vi "Host API Example.vi"() -> ()   [LabVIEW 2013]
uses:
  Shared/Types/Update Parameters Message.ctl
  Shared/Types/Get Settings Message.ctl
  Shared/Types/Gain Schedule.ctl
  Host API/PID Control Host API.lvlib
  Shared/Control Addon Shared.lvlib
panel:
  out "Timed Out?":bool
  out "Settings":T1
  in  "Parameters":T3
  in  "Apply":bool
  in  "Stop":bool
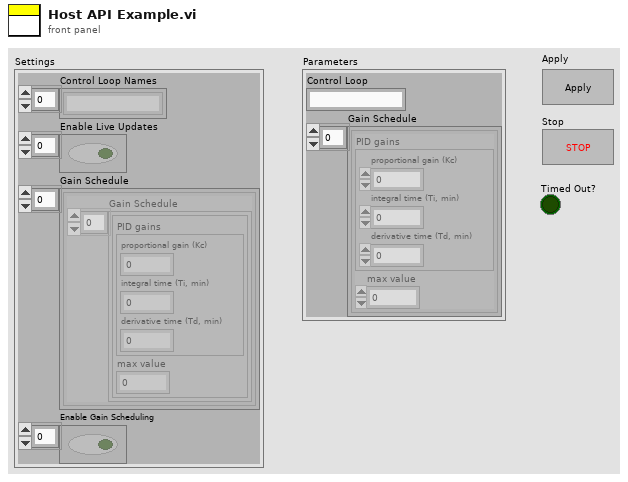
[diagram p1: front panel]
types:
  T1 = typedef "Control Addon Shared.lvlib/Get Settings Message.ctl" = cluster{"Control Loop Names":string[], "Enable Live Updates":bool[], "Gain Schedule":T2[], "Enable Gain Scheduling":bool[]}
  T2 = typedef "Control Addon Shared.lvlib/Gain Schedule.ctl" = cluster{"Gain Schedule":cluster{"PID gains":cluster{"proportional gain (Kc)":dbl, "integral time (Ti, min)":dbl, "derivative time (Td, min)":dbl}, "max value":dbl}[]}
  T3 = typedef "Control Addon Shared.lvlib/Update Parameters Message.ctl" = cluster{"Control Loop":string, "Gain Schedule":cluster{"PID gains":cluster{"proportional gain (Kc)":dbl, "integral time (Ti, min)":dbl, "derivative time (Td, min)":dbl}, "max value":dbl}[]}
  T4 = typedef "Control Addon Shared.lvlib/stm_TCP Connection Info.ctl" = cluster{"connection ID":refnum<k5>, "Meta data":T5[]}
  T5 = typedef "Control Addon Shared.lvlib/stm_MetaDataElement.ctl" = string
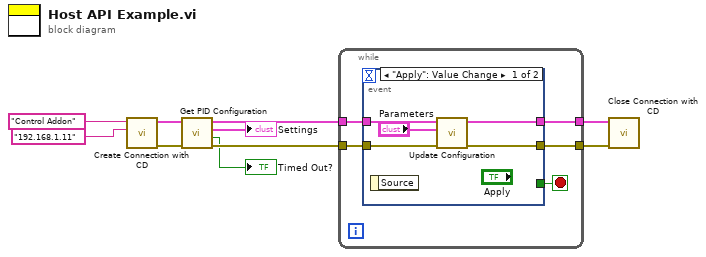
[diagram p0: block diagram]
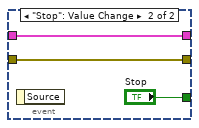
[diagram p2: hidden frame]
diagram:
  n1 = call "Create Connection with CD.vi"("IP Address"="192.168.1.11", "TCP Service"="Control Addon") -> ("error out"=w10:errorcluster, "Connection Info Out"=w3:T4)  [unwired: 8 in]
  n2 = call "Get PID Configuration.vi"("error in (no error)"=w10, "Connection Info"=w3) -> ("error out"=w8:errorcluster, "Timed Out?"=→"Timed Out?":bool, "Settings"=→"Settings":T1, "Connection Info"=w9:T4)  [unwired: 6 in]
  n3 = while {
    tunnel: w9 -> [w15]
    tunnel: w8 -> [w14]
    tunnel: [w13] -> w7
    tunnel: [w12] -> w6
    stop <- w11 stop-if-true
    n4 = event shown="[0] \"Apply\": Value Change" {
      selector: _ -> [_ _]
      dyn-events: _ -> [_ _]
      timeout: _ -> [_ _]
      tunnel: w15 -> [w20 w21]
      tunnel: w14 -> [w19 w22]
      tunnel: [w18 w22] -> w13
      tunnel: [w17 w21] -> w12
      tunnel: [_ "Stop"] -> w11
      event "Apply": Value Change {
        n5 = event-data() -> ()  [unwired: 1 in, 1 out]
        n6 = call "Update Configuration.vi"("error in (no error)"=w19, "Parameters"="Parameters", "Connection Info"=w20) -> ("error out"=w18:errorcluster, "Connection Info"=w17:T4)  [unwired: 5 in, 2 out]
      }
      event "Stop": Value Change {
        n7 = event-data() -> ()  [unwired: 1 in, 1 out]
      }
    }
  }
  n8 = call "Close Connection with CD.vi"("error in"=w7, "Connection Info"=w6) -> ()  [unwired: 9 in, 1 out]
